vi "IDS_GetDllVersion.vi"(8 "error in (no error)":errorcluster, 11 "deviceHandle":i32) -> (0 "error out":errorcluster, 2 "DLL version out":string, 3 "deviceHandle out":i32)   [LabVIEW 2016]
panel:
  in  "version":string
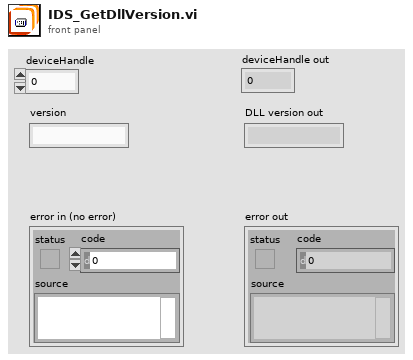
[diagram p1: front panel]
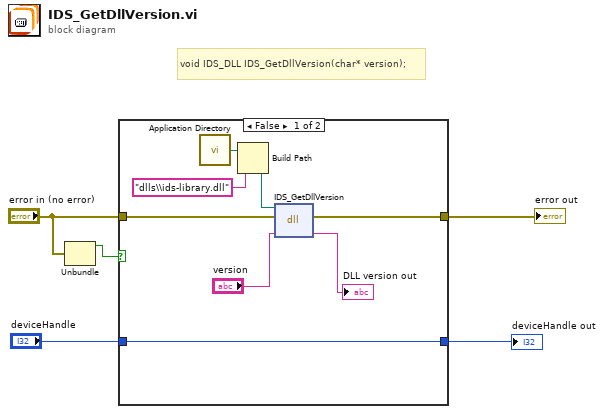
[diagram p0: block diagram]
diagram:
  # "void IDS_DLL IDS_GetDllVersion(char* version);"
  n1 = Unbundle("error in (no error)") -> ("status"=w1:bool)  [unwired: 2 out]
  n2 = case shown="False" w1 {
    tunnel: [w9 w15] -> w5
    tunnel: "error in (no error)" -> [w11 w15]
    tunnel: "deviceHandle" -> [w10 w14]
    tunnel: [w10 w14] -> w3
    frame False {
      n3 = call <vilib>:"Application Directory.vi"() -> ("Application Directory"=w8:path)
      n4 = Build Path(base path=w8, name or relative path="dlls\\ids-library.dll" ("ipAddress")) -> (appended path=w6:path)
      n5 = dll-call lib="C:/Users/matheus/Desktop/LabVIEW_Draft_V1.6.0/dlls/ids-library.*" fn="IDS_GetDllVersion"(path in=w6, error in=w11, "version"="version") -> (error out=w9:errorcluster, "version"=→"DLL version out":string)  [unwired: 2 in, 1 out]
    }
    frame True {
    }
  }
  "error out" <- w5
  "deviceHandle out" <- w3
